vi "Tag Autocomplete Test Panel.vi"() -> ()   [LabVIEW 2020]
panel:
  out "AutoComplete":string[](array[string])
  in  "Tag":string
  in  "Quit":bool
  in  "Tags":string[](array[string])=["test", "testing", "Tester", "Apple", "appeal", "annoy", "lead", "Leed", "Lard", "Lean", "learn", "yo", "yoyo", "You", "your", "yours", "cat", "came", "couple", "001", "02", "0101", "123", "45", "65", "87", "86", "83", "99", "91"]
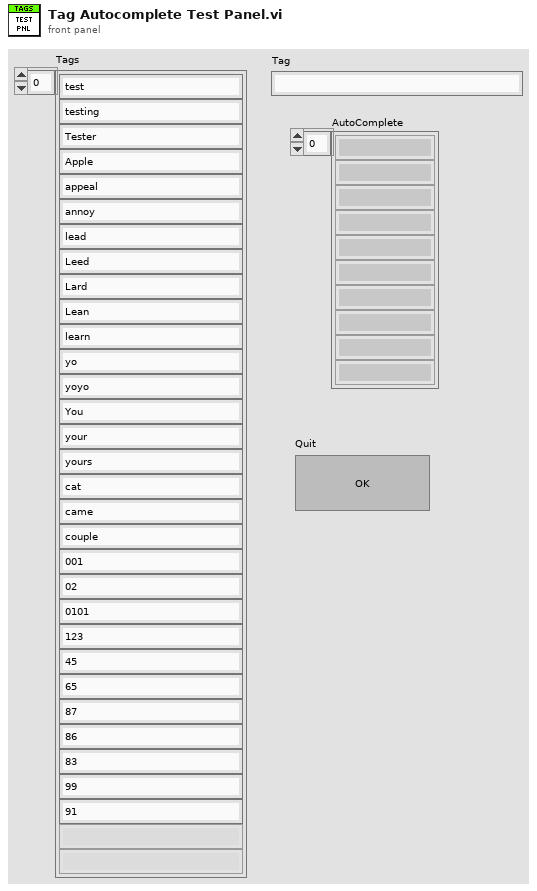
[diagram p1: front panel]
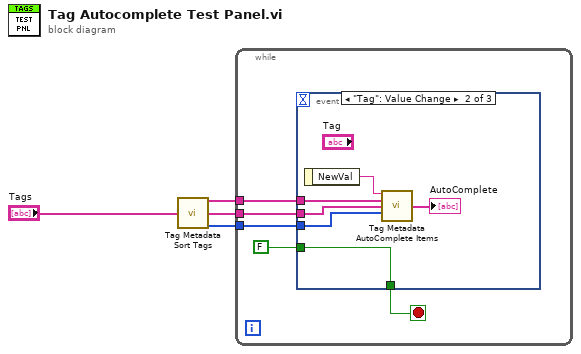
[diagram p0: block diagram]
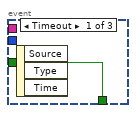
[diagram p2: hidden frame]
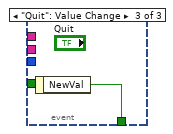
[diagram p3: hidden frame]
diagram:
  n1 = call "Tag Metadata Sort Tags.vi"("Tags"="Tags") -> ("Sorted Tags"=w4:string[], "First Letters"=w3:string[], "Letter Indicies"=w2:i32[])  [unwired: 12 in]
  n2 = while {
    tunnel: w3 -> [w7]
    tunnel: w2 -> [w6]
    tunnel: w4 -> [w5]
    stop <- w9 stop-if-true
    n3 = event shown="[1] \"Tag\": Value Change" {
      selector: _ -> [_ _ _]
      dyn-events: _ -> [_ _ _]
      timeout: _ -> [_ _ _]
      tunnel: [w10 w16 w17] -> w9
      tunnel: FALSE -> [w10 w16 _]
      tunnel: w7 -> [_ w13 _]
      tunnel: w6 -> [_ w12 _]
      tunnel: w5 -> [_ w14 _]
      event Timeout {
        n4 = event-data() -> ()  [unwired: 1 in, 3 out]
      }
      event "Tag": Value Change {
        n5 = event-data() -> ("NewVal"=w15:string)  [unwired: 1 in]
        n6 = call "Tag Metadata AutoComplete Items.vi"("Input String"=w15, "Sorted Tags"=w14, "First Letters"=w13, "Letter Indicies"=w12) -> ("AutoComplete"=→"AutoComplete":string[])  [unwired: 11 in]
      }
      event "Quit": Value Change {
        n7 = event-data() -> ("NewVal"=w17:bool)  [unwired: 1 in]
      }
    }
  }
